vi "Laser_on_CW_pulse_sequence.vi"(1 "Path":path=path "C:/SpinCore/SpinAPI/lib/spinapi64.dll") -> (0 "path out":path=path "C:/SpinCore/SpinAPI/lib/spinapi64.dll")   [LabVIEW 2015]
panel:
  in  "PB Inst 0":T1={"Instruct Data"=0, "Op Code"=0, "Flags"=[TRUE, FALSE, FALSE, FALSE, FALSE, FALSE, FALSE, FALSE, FALSE, FALSE, FALSE, FALSE, FALSE, FALSE, FALSE, FALSE, FALSE, FALSE, FALSE, FALSE, FALSE, FALSE, FALSE, FALSE], "Comments"="MW on", "Time"=5e-05} {"Time" format="%.3p"; "Op Code" items=["Continue", "Stop", "Loop", "End Loop", "JSR", "RTS", "Branch", "Long Delay", "Wait"]}
  in  "PB Inst 1":T1={"Instruct Data"=0, "Op Code"=6, "Flags"=[TRUE, FALSE, FALSE, FALSE, FALSE, FALSE, FALSE, FALSE, FALSE, FALSE, FALSE, FALSE, FALSE, FALSE, FALSE, FALSE, FALSE, FALSE, FALSE, FALSE, FALSE, FALSE, FALSE, FALSE], "Comments"="MW off", "Time"=5e-05} {"Time" format="%.3p"; "Op Code" items=["Continue", "Stop", "Loop", "End Loop", "JSR", "RTS", "Branch", "Long Delay", "Wait"]}
  # "1"
  # "2"
  # "3"
  # "4"
  # "5"
  # "6"
  # "7"
  # "8"
  # "9"
  # "10"
  # "11"
  # "12"
  # "13"
  # "14"
  # "15"
  # "16"
  # "17"
  # "18"
  # "19"
  # "20"
  # "21"
  # "22"
  # "23"
  # "24"
  # "1"
  # "2"
  # "3"
  # "4"
  # "5"
  # "6"
  # "7"
  # "8"
  # "9"
  # "10"
  # "11"
  # "12"
  # "13"
  # "14"
  # "15"
  # "16"
  # "17"
  # "18"
  # "19"
  # "20"
  # "21"
  # "22"
  # "23"
  # "24"
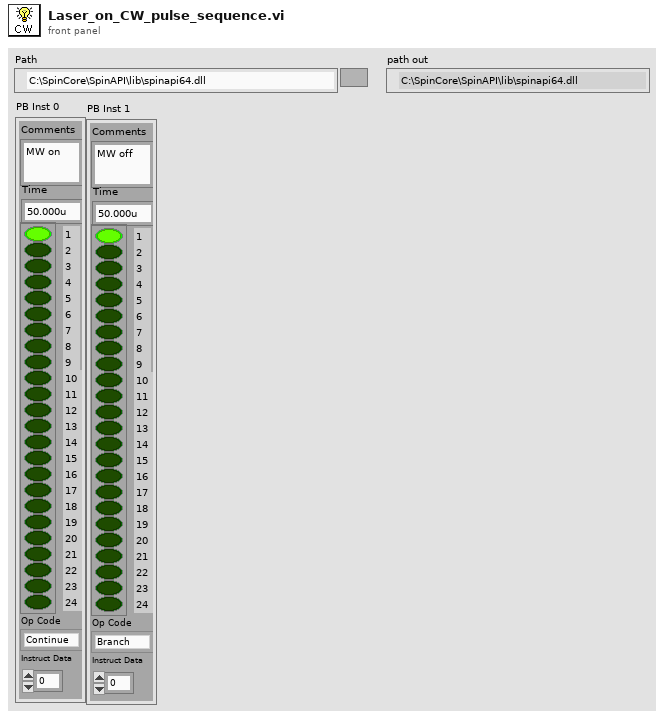
[diagram p1: front panel]
types:
  T1 = cluster{"Instruct Data":i32, "Op Code":i32, "Flags":bool[], "Comments":string, "Time":dbl}
  T2 = enum16{"Pulse Program", "Frequency Registers", "TX Phase Registers", "RX Phase Registers"}
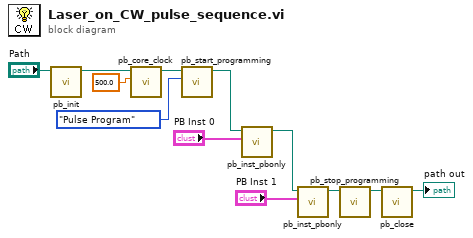
[diagram p0: block diagram]
diagram:
  n1 = call "pb_init.vi"("path in"="Path") -> ("path out"=w5:path)  [unwired: 9 in, 1 out]
  n2 = call "pb_core_clock.vi"("clock_freq (MHz)"=500.0, "path in"=w5) -> ("path out"=w11:path)  [unwired: 8 in, 1 out]
  n3 = call "pb_start_programming.vi"("Device"=T2."Pulse Program", "path in"=w11) -> ("path out"=w8:path)  [unwired: 8 in, 1 out]
  n4 = call "pb_inst_pbonly.vi"("PB Instruction"="PB Inst 0", "path in"=w8) -> ("path out"=w7:path)  [unwired: 8 in, 1 out]
  n5 = call "pb_inst_pbonly.vi"("PB Instruction"="PB Inst 1", "path in"=w7) -> ("path out"=w6:path)  [unwired: 8 in, 1 out]
  n6 = call "pb_stop_programming.vi"("path in"=w6) -> ("path out"=w3:path)  [unwired: 9 in, 1 out]
  n7 = call "pb_close.vi"("path in"=w3) -> ("path out"=→"path out":path)  [unwired: 9 in, 1 out]
